vi "Read Dew Point DBL.vi"(8 "error in":errorcluster, 10 "Source":string, 11 "Virtual NEO480 in":refnum<class "Virtual NEO480.lvclass">) -> (0 "error out":errorcluster, 1 "Time Stamp":timestamp format="%<%x %.3X>T", 2 "Dew Point":dbl, 3 "Virtual NEO480 out":refnum<class "Virtual NEO480.lvclass">)   [LabVIEW 2024, in "Virtual NEO480.lvclass"]
uses:
  Virtual NEO480.lvclass
  Virtual NEO480.lvclass/Virtual NEO480.ctl
  Source/DBC Communicator/DBC Communicator.lvclass
  Source/Action Point/Action Point.lvclass
  Source/Interfaces/ILog Data/ILog Data.lvclass
  D:/git/HAL/Source/Action Point/Action Point.lvclass
  D:/git/HAL/Source/Interfaces/IVirtual Instrument/IVirtual Instrument.lvclass
  D:/git/HAL/Source/Interfaces/IClose/IClose.lvclass
  D:/git/HAL/Source/Interfaces/IHas Configuration/IHas Configuration.lvclass
  D:/git/HAL/Source/Interfaces/IInitialize/IInitialize.lvclass
  D:/git/HAL/Source/Interfaces/IRunnable/IRunnable.lvclass
  D:/git/HAL/HAL-Devices/Source/Virtual Instruments/Virtual NEO480/Virtual NEO480.lvclass
  D:/git/HAL/Source/Interfaces/IRead Dew Point/IRead Dew Point.lvclass
  D:/git/HAL/Source/Interfaces/IRead H2O Concentration/IRead H2O Concentration.lvclass
  D:/git/HAL/Source/Interfaces/IRead Humidity/IRead Humidity.lvclass
  D:/git/HAL/Source/Interfaces/IReadPressure/IRead Pressure.lvclass
  D:/git/HAL/Source/Interfaces/IRead Temperature/IRead Temperature.lvclass
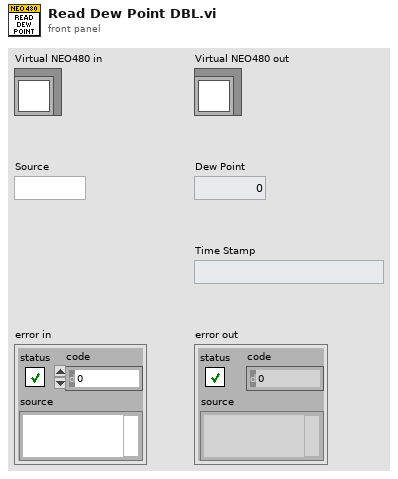
[diagram p1: front panel]
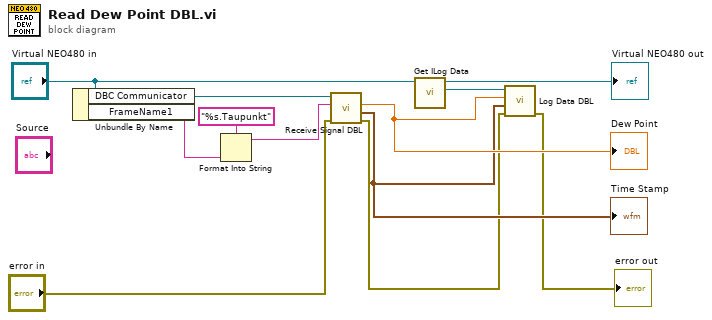
[diagram p0: block diagram]
diagram:
  n1 = Unbundle By Name("Virtual NEO480 in") -> ("DBC Communicator"=w10:refnum<class "DBC Communicator.lvclass">, "FrameName1"=w11:string)
  n2 = Format Into String(format string="%s.Taupunkt", w11) -> (resulting string=w9:string)  [unwired: 2 in, 1 out]
  n3 = call "Receive Signal DBL.vi"("error in"="error in", "Signal Name"=w9, "DBC Communication in"=w10) -> ("error out"=w2:errorcluster, "Time Stamp"=w3:timestamp, "Value"=w4:dbl)  [unwired: 5 in, 1 out]
  "Dew Point" <- w4
  "Time Stamp" <- w3
  n4 = call "Get ILog Data.vi"("Action Point in"="Virtual NEO480 in") -> ("ILog Data"=w7:refnum<class "ILog Data.lvclass">, "Action Point out"=→"Virtual NEO480 out":refnum<class "Virtual NEO480.lvclass">)  [unwired: 9 in]
  n5 = call-dynamic "Log Data DBL.vi"("error in"=w2, "Time Stamp"=w3, "Data"=w4, "IDataLogger in"=w7) -> ("error out"=→"error out":errorcluster)  [unwired: 6 in, 1 out]
